vi "RT Stop.vi"(8 "error in (no error)":errorcluster, 11 "1553 Unit Test in":refnum<class "Remote Terminal.lvclass">) -> (0 "error out":errorcluster, 3 "1553 Unit Test out":refnum<class "Remote Terminal.lvclass">)   [LabVIEW 2020, in "Unit Tests.lvlib" / "Remote Terminal.lvclass"]
uses:
  Remote Terminal.lvclass
  Remote Terminal.lvclass/Remote Terminal.ctl
  <vilib>/addons/_JKI Toolkits/Caraya/classes/Assert/Assert True.vi
  1553 Session/1553 Session.lvclass
  Dependencies/FPGA Interface/FPGA Interface.lvclass
  <vilib>/addons/_JKI Toolkits/Caraya/classes/Assert/Assert.lvclass
  <vilib>/addons/_JKI Toolkits/Caraya/classes/Test/Test.lvclass
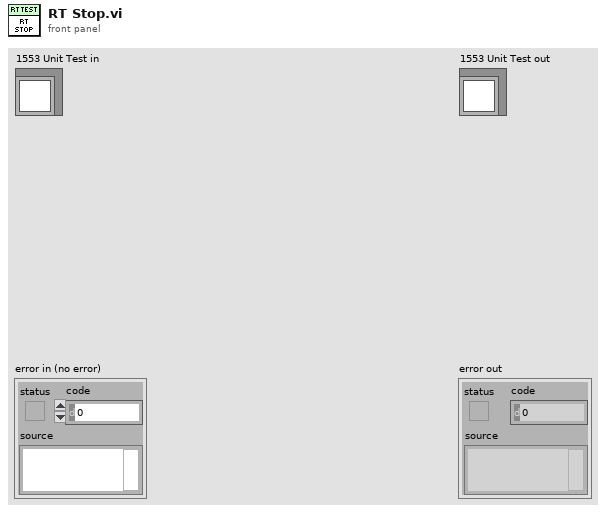
[diagram p1: front panel]
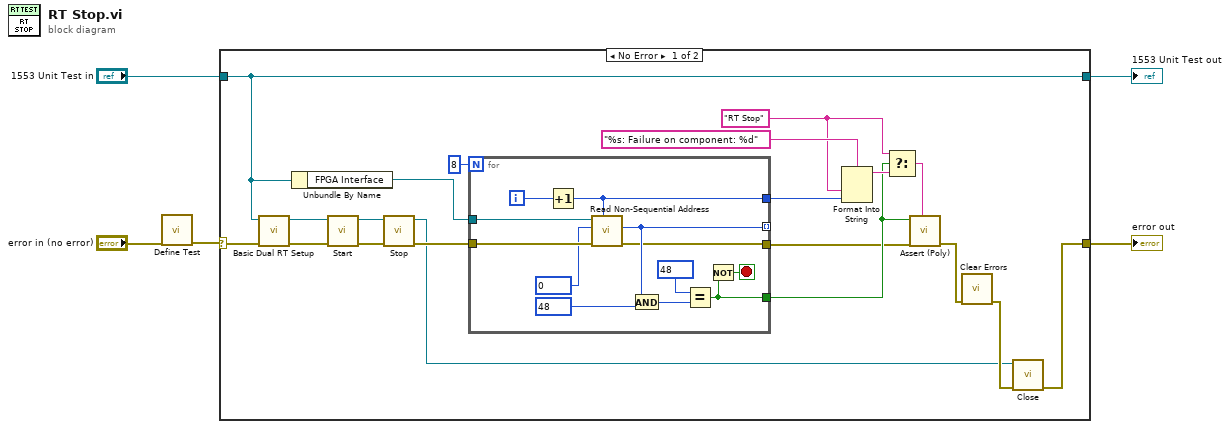
[diagram p0: block diagram]
diagram:
  n1 = call <vilib>:"Define Test.vi"("error in (no error)"="error in (no error)") -> ("error out"=w2:errorcluster)  [unwired: 9 in, 1 out]
  n2 = case shown="No Error" w2 {
    selector: w2 -> [w21 w39]
    tunnel: [w7 w39] -> w5
    tunnel: [w10 w38] -> w3
    tunnel: "1553 Unit Test in" -> [w10 w38]
    frame No Error {
      w22 = "RT Stop" ("custom report message (\"\")")
      n3 = call "Basic Dual RT Setup.vi"("error in (no error)"=w21, "1553 Unit Test in"=w10) -> ("error out"=w18:errorcluster, "1553 Session out"=w11:refnum<class "1553 Session.lvclass">)  [unwired: 8 in]
      n4 = Unbundle By Name(w10) -> ("FPGA Interface"=w15:refnum<class "FPGA Interface.lvclass">)
      n5 = call-dynamic "Start.vi"("error in (no error)"=w18, "1553 Board in"=w11) -> ("error out"=w19:errorcluster, "1553 Board out"=w20:refnum<class "1553 Session.lvclass">)  [unwired: 8 in]
      n6 = call-dynamic "Stop.vi"("error in (no error)"=w19, "1553 Board in"=w20) -> ("error out"=w16:errorcluster, "1553 Board out"=w6:refnum<class "1553 Session.lvclass">)  [unwired: 8 in]
      n7 = for {
        N: 8 -> [_]
        tunnel: w15 -> [w37]
        tunnel: w16 -> [w35]
        tunnel: [w27] -> w13
        tunnel: [w30] -> w14
        tunnel: [w29] -> _ mode=indexing
        tunnel: [w26] -> w12
        i -> [w36]
        stop <- w28 stop-if-true
        n8 = Increment(x=w36) -> (x+1=w30:i32)
        n9 = call-dynamic "Read Non-Sequential Address.vi"("Target IC (1-8)"=w30, "error in (no error)"=w35, "Address"=u16 0, "FPGA Interface in"=w37) -> ("error out"=w26:errorcluster, "Data"=w29:u16)  [unwired: 6 in]
        n10 = And(x=w29, y=u16 48) -> (x .and. y?=w31:u16)
        n11 = Equal?(x=u16 48, y=w31) -> (x = y?=w27:bool)
        n12 = Not(x=w27) -> (.not. x?=w28:bool)
      }
      n13 = Format Into String(format string="%s: Failure on component: %d" ("custom report message (\"\")"), w22, w14) -> (resulting string=w24:string)  [unwired: 2 in, 1 out]
      n14 = Select(t=w22, s=w13, f=w24) -> (s? t:f=w23:string)
      n15 = call-poly <vilib>:"Assert (Poly).vi"("Label"=w23, "error in (no error)"=w12, "True?"=w13) -> ("error out"=w9:errorcluster)  [unwired: 7 in, 1 out]
      n16 = call <vilib>:"Clear Errors.vi"("error in (no error)"=w9) -> ("error out"=w8:errorcluster)  [unwired: 5 in, 1 out]
      n17 = call-dynamic "Close.vi"("error in (no error)"=w8, "1553 Board in"=w6) -> ("error out"=w7:errorcluster)  [unwired: 9 in]
    }
    frame Error {
    }
  }
  "error out" <- w5
  "1553 Unit Test out" <- w3
